vi "Sub Super Duper_7_26_12a_JW.vi"(0 "VISA resource name":refnum<visa-resource-name>="GPIB0::17::INSTR", 1 "Sample Properties:":T6 {"Date Created" format="%<%Y/%m/%d>T"}, 2 "TRF Cluster":T7={"Step 4"=-38.0, "# of Loops"=1.0, "Transfer 2"=FALSE, "Start 4"=-2.0, "Total Points 2"=2, "Start 3"=40.0, "Stop 2"=-40.0, "Step 3"=-1.0, "Loop Step"=0.0, "Integration Time 3"=0, "Loop Wait"=0.0, "First Step"=0.0} {"Loop Wait" format="%<%H:%M:%S>t"; "Integration Time 3" scale=0.0..2.0; "Step 3" format="%.2f"; "Stop 2" format="%.2f"; "Start 3" format="%.2f"; "Start 4" format="%.2f"; "Step 4" format="%.2f"}, 3 "TSP Cluster":T8={"Transport"=FALSE, "Start 2"=0.0, "Stop 3"=-60.0, "Step 2"=-1.0, "Start"=0.0, "Step"=-10.0, "Total Points"=7, "Integration Time"=0} {"Integration Time" scale=0.0..2.0; "Step" format="%.2f"; "Start" format="%.2f"; "Step 2" format="%.2f"; "Stop 3" format="%.2f"; "Start 2" format="%.2f"}, 4 "Compliance Cluster":T3={"Var1 sweep settings"={"sweep spacing (linear: 0)"=0, "sweep mode"=FALSE, "compliance (V)"=100.0, "compliance (A)"=0.001}, "Var1 sweep settings 2"={"sweep spacing (linear: 0)"=0, "sweep mode"=FALSE, "compliance (V)"=100.0, "compliance (A)"=0.001}, "Var2 step settings 2"={"compliance (A)"=0.001, "compliance (V)"=100.0}, "Var2 step settings"={"compliance (A)"=0.001, "compliance (V)"=100.0}} {"Var2 step settings"."compliance (V)" format="%.2f"; "Var2 step settings"."compliance (A)" format="%^.2e"; "Var2 step settings 2"."compliance (V)" format="%.2f"; "Var2 step settings 2"."compliance (A)" format="%^.2e"; "Var1 sweep settings 2"."compliance (A)" format="%^.2e"; "Var1 sweep settings 2"."compliance (V)" format="%.2f"; "Var1 sweep settings 2"."sweep spacing (linear: 0)" items=["linear", "log 10", "log 25", "log 50"]; "Var1 sweep settings"."compliance (A)" format="%^.2e"; "Var1 sweep settings"."compliance (V)" format="%.2f"; "Var1 sweep settings"."sweep spacing (linear: 0)" items=["linear", "log 10", "log 25", "log 50"]}, 5 "error in":errorcluster, 6 "Saved Folder:":path=path "C:/1DATA/2011", 7 "Wait Cluster":T2 {"Wait Time (s)" format="%.1g"; "Wait Countdown" format="%<%H:%M:%S%1u>t"}, 9 "Stop \nCountdown":bool, 11 "Loop Count":dbl) -> (8 "Status Indicator":bool, 10 "Vt Cluster":T1 {"Id Max" format="%.3g"; "Vt Max" format="%.3g"; "Vt Min" format="%.3g"; "Vt Ratio" format="%.3g"}, 13 "Raw Graph":cluster{dbl[], dbl[]}[](graph), 14 "VISA resource name out":refnum<visa-resource-name>, 15 "TRF Path":path, 16 "TSP Path":path, 17 "Graph Cluster":T4, 18 "Char Cluster":T5 {"Mobility-Lin" format="%#_4e"; "On/Off" format="%#_4e"; "Mobility-Sat" format="%#_4e"}, 19 "error out":errorcluster)   [LabVIEW 2011]
uses:
  <vilib>/Platform/TimedLoop/XDataNode/wakeup.ctl
  <vilib>/Platform/TimedLoop/XDataNode/XDNodeRunTimeDep.lvlib
  <vilib>/Platform/TimedLoop/XDataNode/nitl_modes.ctl
  <vilib>/Platform/TimedLoop/XDataNode/timing_clust.ctl
  <vilib>/Platform/TimedLoop/XDataNode/XDataNode.xnode
panel:
  in  "Transport Temp":cluster{"trace":dbl[], "trace":dbl[]}(graph)
  in  "Graph":cluster{dbl[], "trace":dbl[]}[](graph) caption="Transfer"
  # "Vg Sweep"
  # "Vd Step"
  # "Loops and Integration Time"
  # "Device Characteristics"
  # "Sample Properties:"
  # "%"
  # "nm"
  # "Device Properties:"
  # "um"
  # "um"
  # "Vg Step"
  # "Vd Step"
  # "Integration Time"
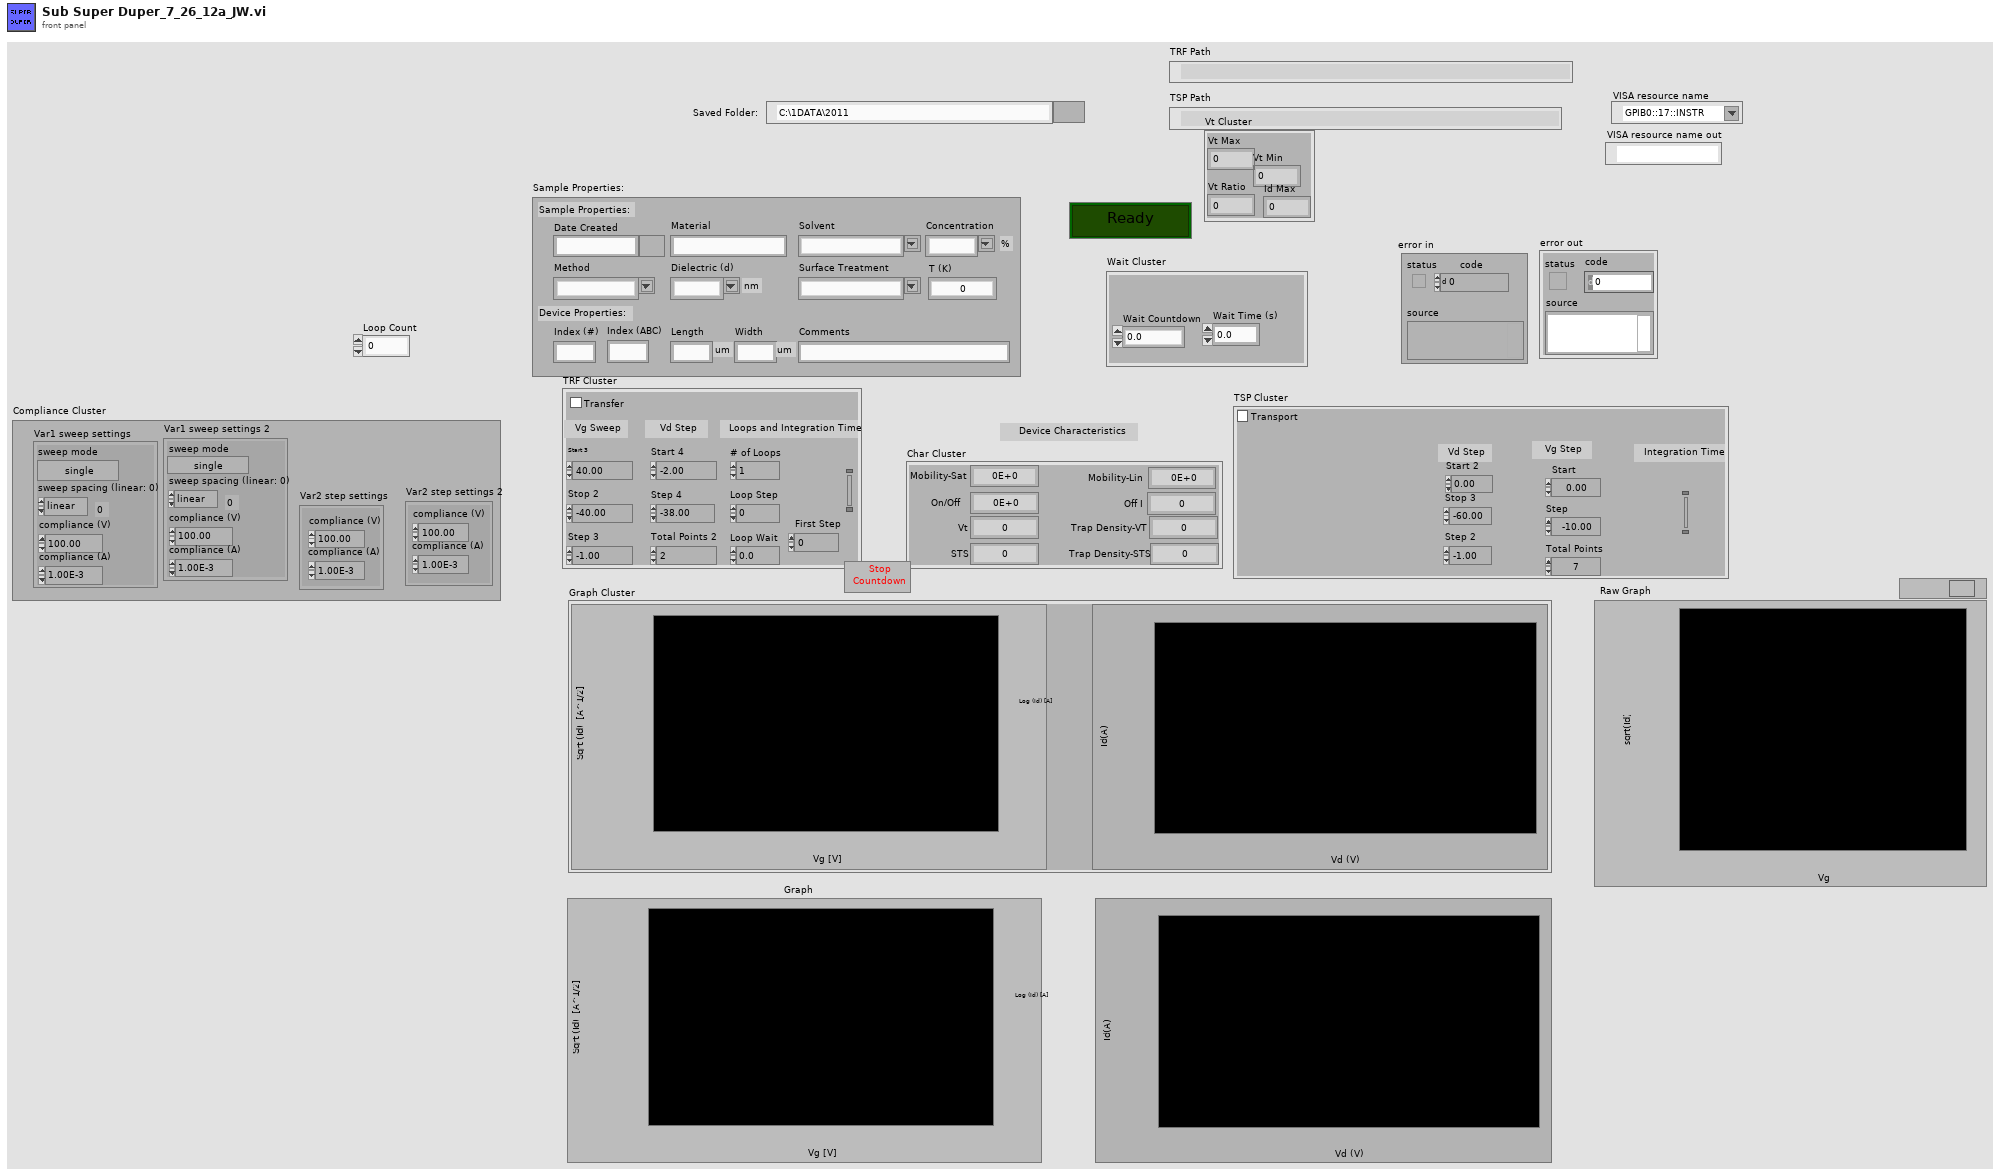
[diagram p1: front panel]
types:
  T1 = cluster{"Vt Max":i32, "Vt Min":i32, "Vt Ratio":i32, "Id Max":i32}
  T2 = cluster{"Wait Countdown":dbl, "Wait Time (s)":dbl}
  T3 = cluster{"Var1 sweep settings":cluster{"sweep spacing (linear: 0)":u16, "sweep mode":bool, "compliance (V)":dbl, "compliance (A)":dbl}, "Var1 sweep settings 2":cluster{"sweep spacing (linear: 0)":u16, "sweep mode":bool, "compliance (V)":dbl, "compliance (A)":dbl}, "Var2 step settings 2":cluster{"compliance (A)":dbl, "compliance (V)":dbl}, "Var2 step settings":cluster{"compliance (A)":dbl, "compliance (V)":dbl}}
  T4 = cluster{"Transfer":cluster{dbl[], "trace":dbl[]}[], "Transport":cluster{"trace":dbl[], "trace":dbl[]}}
  T5 = cluster{"Mobility-Sat":dbl, "Mobility-Lin":dbl, "On/Off ":dbl, "Off I":dbl, "Vt":dbl, "STS":dbl, "Trap Density-VT":dbl, "Trap Density-STS":dbl}
  T6 = cluster{"Date Created":timestamp, "Material":string, "Solvent":string, "Concentration":string, "Method":string, "Dielectric (d)":string, "Index (#)":string, "Index (ABC)":string, "Length":string, "Width":string, "Surface Treatment":string, "Comments":string, "T (K)":dbl}
  T7 = cluster{"Step 4":dbl, "# of Loops":dbl, "Transfer 2":bool, "Start 4":dbl, "Total Points 2":u16, "Start 3":dbl, "Stop 2":dbl, "Step 3":dbl, "Loop Step":dbl, "Integration Time 3":u32, "Loop Wait":dbl, "First Step":dbl}
  T8 = cluster{"Transport":bool, "Start 2":dbl, "Stop 3":dbl, "Step 2":dbl, "Start":dbl, "Step":dbl, "Total Points":u16, "Integration Time":u32}
  T9 = typedef "XDNodeRunTimeDep.lvlib/timing_clust.ctl" = cluster{"Expected End [f-1]":u64, "Actual End [f-1]":u64, "Finished Late? [f-1]":bool, "Expected End [i-1]":u64, "Actual End [i-1]":u64, "Finished Late? [i-1]":bool, "Expected Start [i]":u64, "Actual Start [i]":u64, "Expected Start [f]":u64, "Actual Start [f]":u64, "Source Name":string, "Structure Name":string, "Period":i64, "Deadline":i64, "Offset":i64, "Start":i64, "Priority":i32, "Timeout":i32, "Mode":T10, "Wakeup Reason":T11, "Error":errorcluster, "Source Type":string, "Secondary Source Type":string, "Global End Time":u64, "Global Start Time":u64, "Frame Duration":u64, "Iteration Duration":u64, "Assigned CPU":i32, "I/O Scan Engine Mode":u32}
  T10 = typedef "XDNodeRunTimeDep.lvlib/nitl_modes.ctl" = enum32{"No Change", "Process missed periods, maintain original phase", "Discard missed periods, maintain original phase", "Process missed periods, ignore original phase", "Discard missed periods, ignore original phase"}
  T11 = typedef "XDNodeRunTimeDep.lvlib/wakeup.ctl" = enum32{"Normal", "Aborted", "Asynchronous wakeup", "Timing source error", "Timed loop error", "Timeout"}
  T12 = cluster{"sweep spacing (linear: 0)":u16, "sweep mode":bool, "compliance (V)":dbl, "compliance (A)":dbl}
  T13 = cluster{"compliance (A)":dbl, "compliance (V)":dbl}
  T14 = cluster{"Start 3":dbl, "Stop 2":dbl, "Step 3":dbl, "sweep spacing (linear: 0)":u16, "sweep mode":bool, "compliance (V)":dbl, "compliance (A)":dbl}
  T15 = cluster{"compliance (A)":dbl, "compliance (V)":dbl, "Start 4":dbl, "Total Points 2":u16, dbl}
  T16 = cluster{"Vt Max":i32, "Vt Min":i32, "Vt Ratio":i32, "Id Max":dbl}
  T17 = cluster{"Mobility-Sat":dbl, "Mobility-Lin":dbl, "On/Off Current":dbl, "Off I":dbl, "Vt":dbl, "STS":dbl, "Trap Density-VT":dbl, "Trap Density-STS":dbl}
  T18 = cluster{"Start 2":dbl, "Stop 3":dbl, "Step 2":dbl, "sweep spacing (linear: 0)":u16, "sweep mode":bool, "compliance (V)":dbl, "compliance (A)":dbl}
  T19 = cluster{"compliance (A)":dbl, "compliance (V)":dbl, "Start":dbl, "Total Points":u16, "Step":dbl}
  T20 = cluster{"Graph":cluster{dbl[], "trace":dbl[]}[], "Transport Temp":cluster{"trace":dbl[], "trace":dbl[]}}
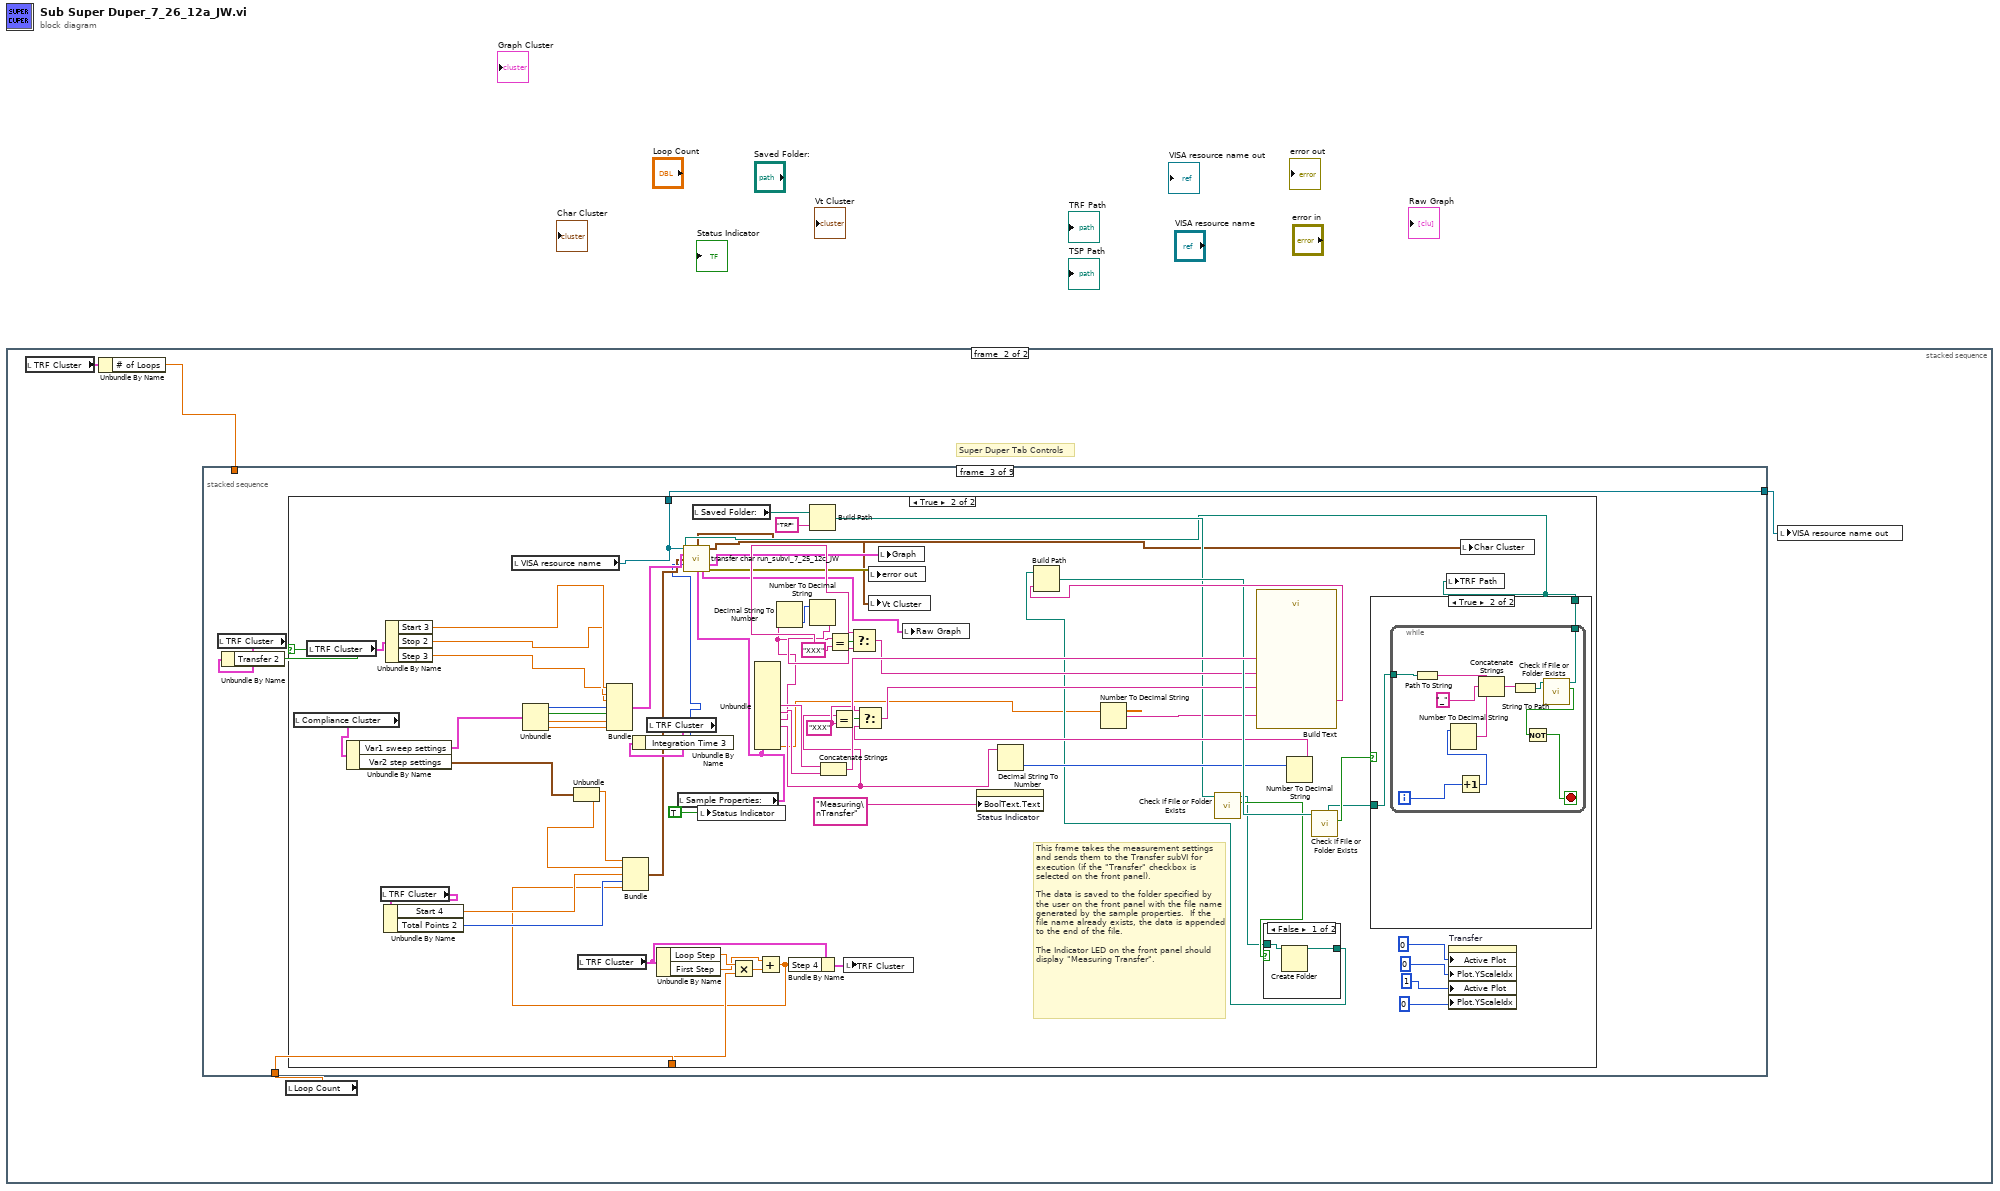
[diagram p0: block diagram]
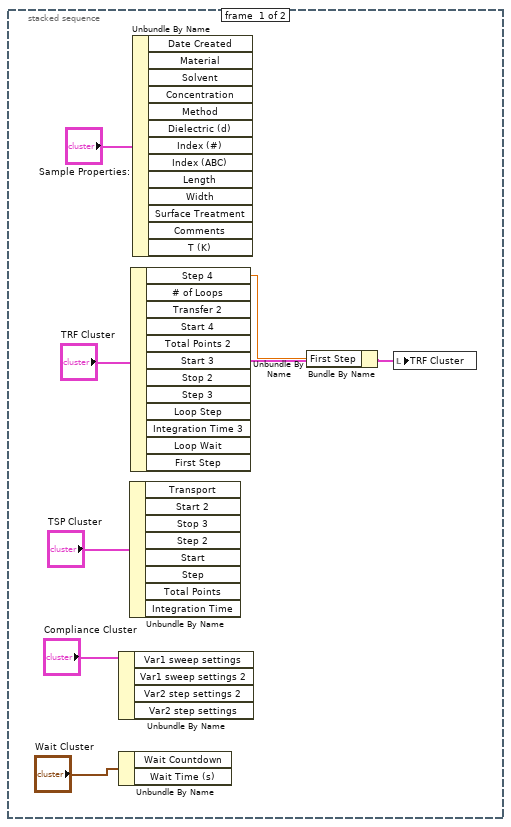
[diagram p2: hidden frame]
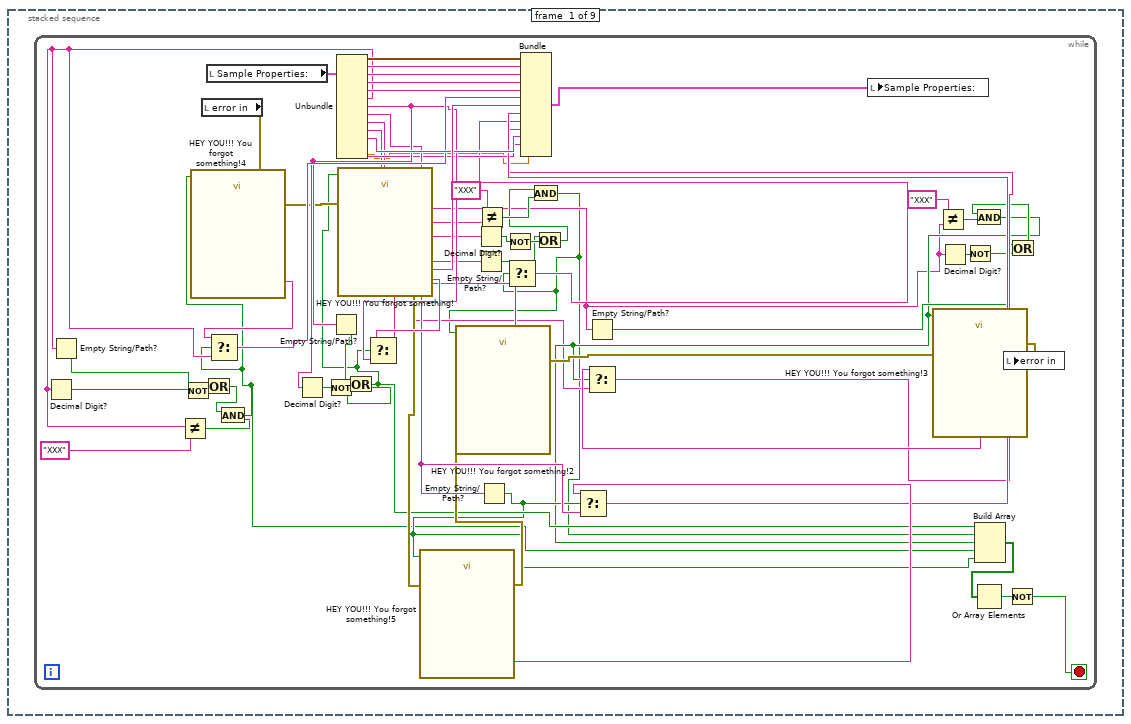
[diagram p3: hidden frame]
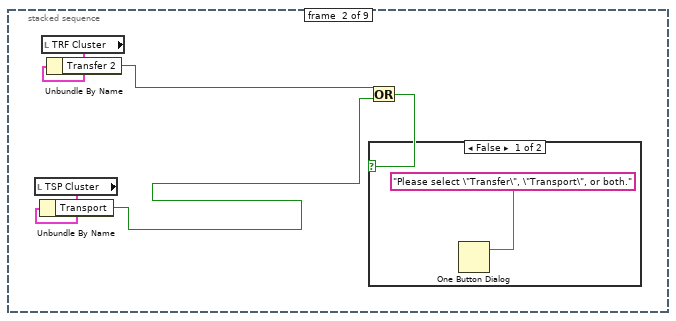
[diagram p4: hidden frame]
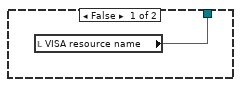
[diagram p6: hidden frame]
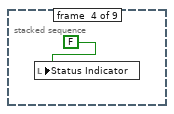
[diagram p9: hidden frame]
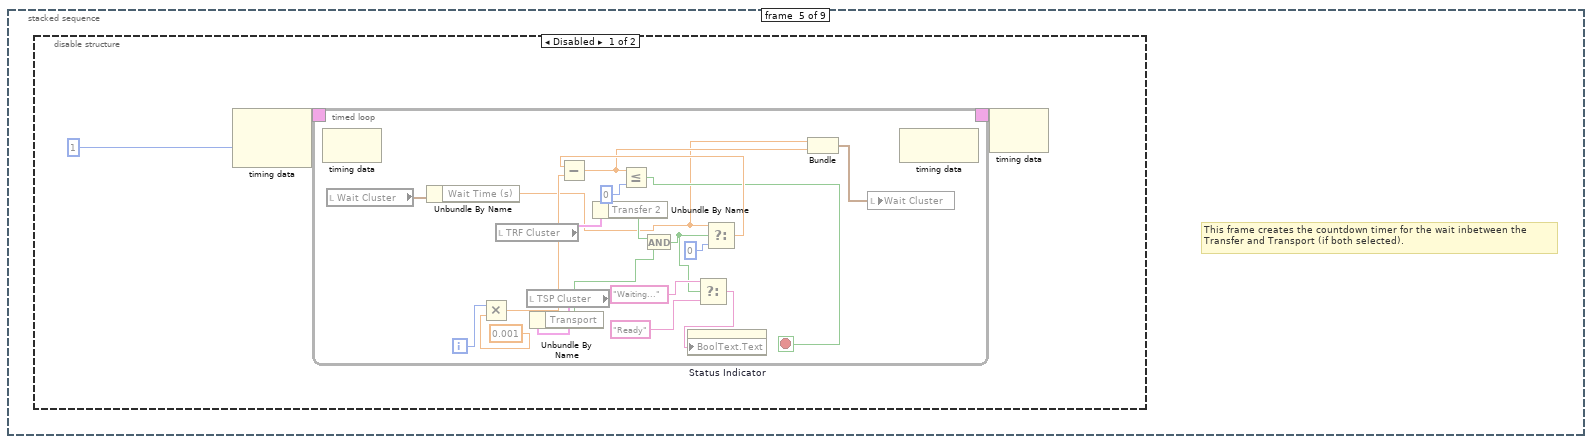
[diagram p10: hidden frame]
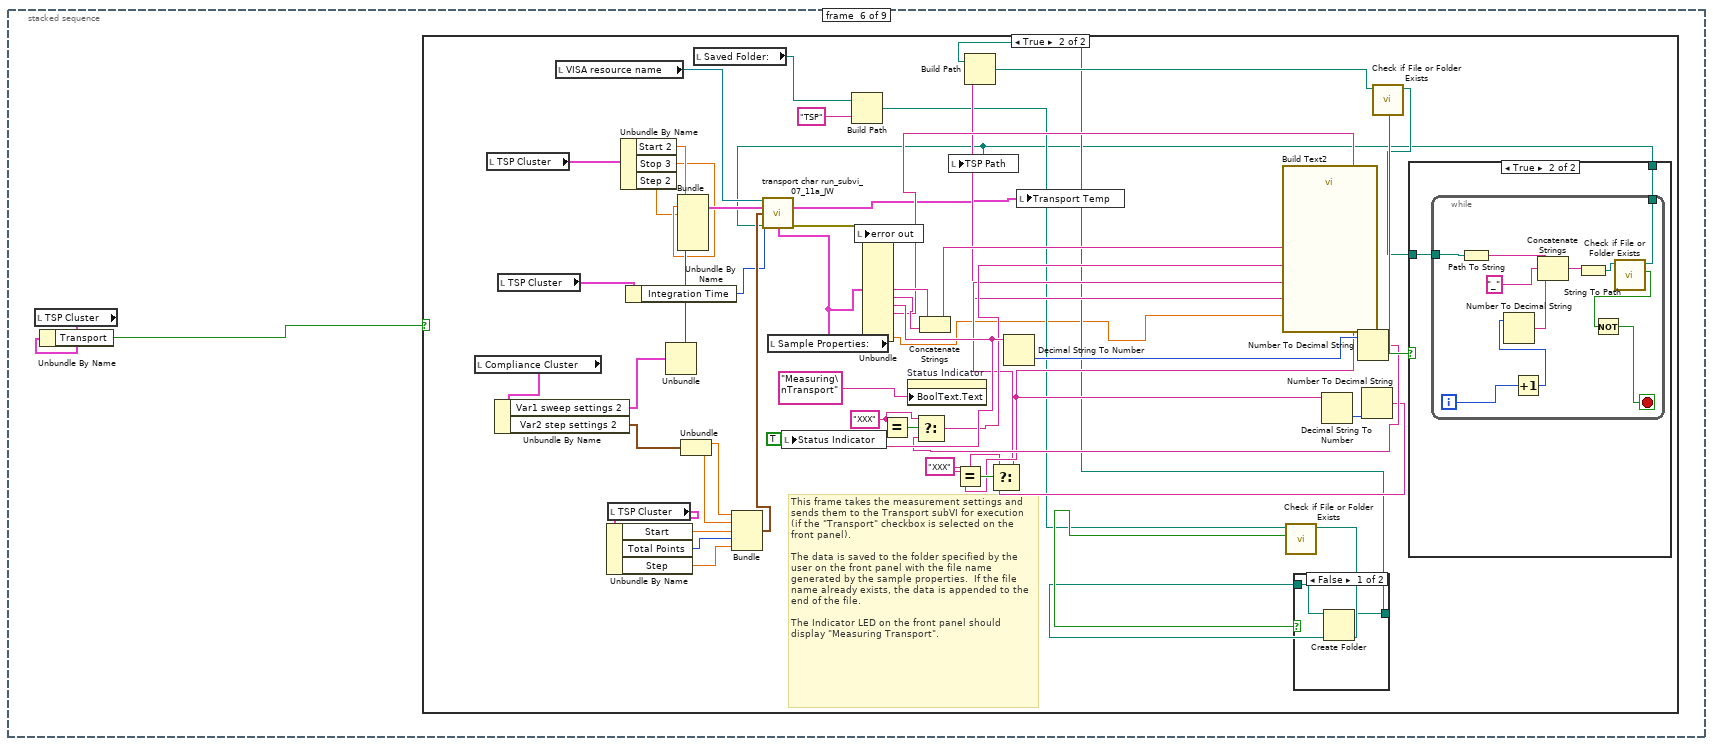
[diagram p12: hidden frame]
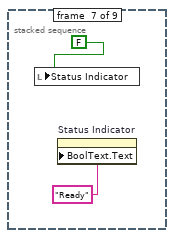
[diagram p16: hidden frame]
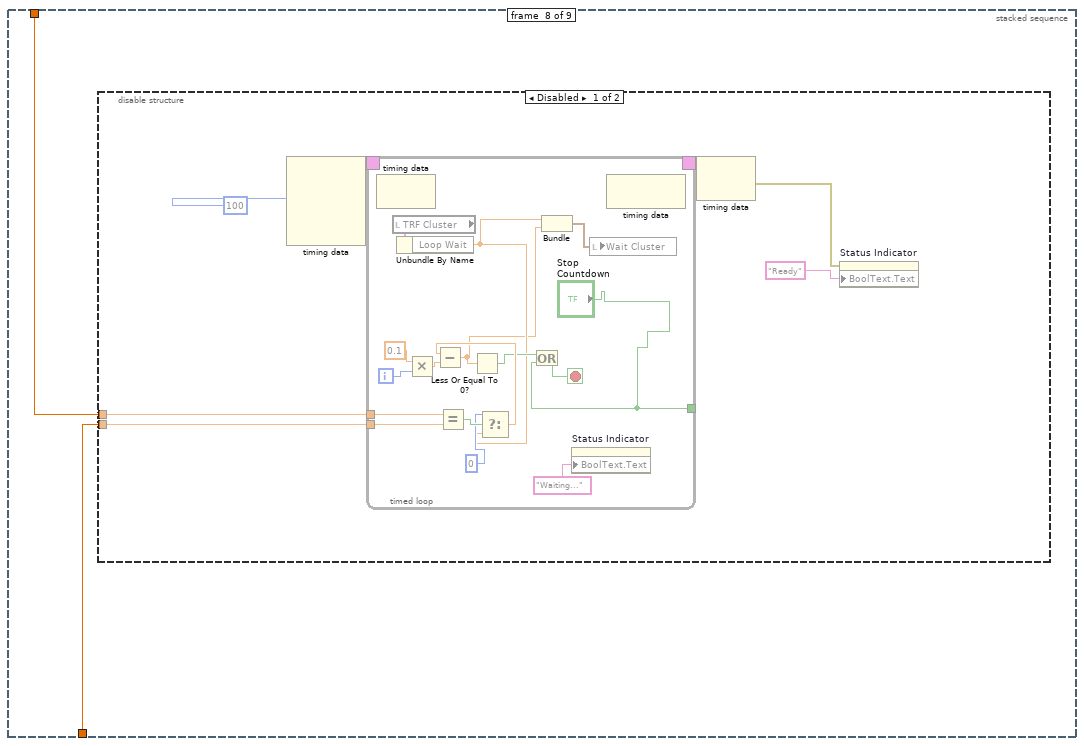
[diagram p17: hidden frame]
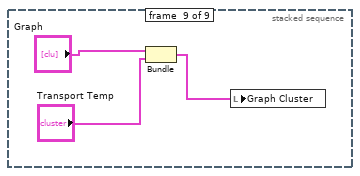
[diagram p19: hidden frame]
diagram:
  n1 = stacked-sequence {
    frame #0 {
      n2 = Unbundle By Name("Compliance Cluster") -> ()  [unwired: 4 out]
      n3 = Unbundle By Name("Wait Cluster") -> ()  [unwired: 2 out]
      n4 = Unbundle By Name("TSP Cluster") -> ()  [unwired: 8 out]
      n5 = Unbundle By Name("TRF Cluster") -> ("Step 4"=w7:dbl)  [unwired: 11 out]
      n6 = Unbundle By Name("Sample Properties:") -> ()  [unwired: 13 out]
      n7 = Bundle By Name(cluster="TRF Cluster", "First Step"=w7) -> (w5:T7)
      n8 = local write "TRF Cluster"(w5) -> ()
    }
    frame #1 {
      # "Super Duper Tab Controls"
      n9 = local read "TRF Cluster"() -> (w11:T7)
      n10 = Unbundle By Name(w11) -> ("# of Loops"=w10:dbl)
      n11 = local read "Loop Count"() -> (w8:dbl)
      n12 = stacked-sequence {
        tunnel: w8 -> [_ _ w81 _ _ _ _ w273 _]
        tunnel: w10 -> [_ _ _ _ _ _ _ w272 _]
        tunnel: [_ _ w78 _ _ _ _ _ _] -> w9
        frame #0 {
          n13 = while {
            stop <- w37 stop-if-true
            n14 = local read "error in"() -> (w43:errorcluster)
            n15 = local read "Sample Properties:"() -> (w66:T6)
            n16 = Unbundle(w66) -> ("Date Created"=w67:timestamp, "Material"=w68:string, "Solvent"=w69:string, "Concentration"=w70:string, "Method"=w71:string, "Dielectric (d)"=w26:string, "Index (#)"=w56:string, "Index (ABC)"=w53:string, "Length"=w21:string, "Width"=w14:string, "Surface Treatment"=w59:string, "Comments"=w51:string, "T (K)"=w12:dbl)
            n17 = Decimal Digit?(1:w26) -> (0:w34:bool)
            n18 = Empty String/Path?(string/path=w26) -> (empty?=w28:bool)
            n19 = Not Equal?(x=w26, y="XXX") -> (x != y?=w25:bool)
            n20 = Not(x=w34) -> (.not. x?=w31:bool)
            n21 = Or(x=w28, y=w31) -> (x .or. y?=w24:bool)
            n22 = And(x=w24, y=w25) -> (x .and. y?=w23:bool)
            n23 = call "HEY YOU!!! You forgot something!4"("Enable"=w23, "error in (no error)"=w43) -> ("Dielectric (d)"=w58:string, "error out"=w42:errorcluster)  [unwired: 15 in, 1 out]
            n24 = Select(t=w58, s=w23, f=w26) -> (s? t:f=w57:string)
            n25 = Decimal Digit?(1:w56) -> (0:w47:bool)
            n26 = Not(x=w47) -> (.not. x?=w46:bool)
            n27 = Empty String/Path?(string/path=w56) -> (empty?=w55:bool)
            n28 = Or(x=w55, y=w46) -> (x .or. y?=w41:bool)
            n29 = call "HEY YOU!!! You forgot something!"("Enable"=w41, "error in (no error)"=w42) -> ("Index (#)"=w65:string, "error out"=w45:errorcluster)  [unwired: 15 in, 1 out]
            n30 = Select(t=w65, s=w41, f=w56) -> (s? t:f=w62:string)
            n31 = Decimal Digit?(1:w21) -> (0:w36:bool)
            n32 = Empty String/Path?(string/path=w21) -> (empty?=w30:bool)
            n33 = Not Equal?(x="XXX", y=w21) -> (x != y?=w20:bool)
            n34 = Empty String/Path?(string/path=w53) -> (empty?=w40:bool)
            n35 = call "HEY YOU!!! You forgot something!5"("Enable"=w40, "error in (no error)"=w45) -> ("Index (ABC)"=w54:string, "error out"=w44:errorcluster)  [unwired: 15 in, 1 out]
            n36 = Not(x=w36) -> (.not. x?=w33:bool)
            n37 = Or(x=w30, y=w33) -> (x .or. y?=w19:bool)
            n38 = And(x=w19, y=w20) -> (x .and. y?=w13:bool)
            n39 = call "HEY YOU!!! You forgot something!2"("Enable"=w13, "error in (no error)"=w44) -> ("Length"=w64:string, "error out"=w61:errorcluster)  [unwired: 15 in, 1 out]
            n40 = Select(t=w64, s=w13, f=w21) -> (s? t:f=w50:string)
            n41 = Select(t=w54, s=w40, f=w53) -> (s? t:f=w52:string)
            n42 = Empty String/Path?(string/path=w14) -> (empty?=w29:bool)
            n43 = Not Equal?(x="XXX", y=w14) -> (x != y?=w18:bool)
            n44 = Decimal Digit?(1:w14) -> (0:w35:bool)
            n45 = Not(x=w35) -> (.not. x?=w32:bool)
            n46 = Or(x=w29, y=w32) -> (x .or. y?=w17:bool)
            n47 = And(x=w17, y=w18) -> (x .and. y?=w16:bool)
            n48 = call "HEY YOU!!! You forgot something!3"("Enable"=w16, "error in (no error)"=w61) -> ("Width"=w63:string, "error out"=w60:errorcluster)  [unwired: 15 in, 1 out]
            n49 = Select(t=w63, s=w16, f=w14) -> (s? t:f=w49:string)
            n50 = Bundle("Date Created"=w67, "Material"=w68, "Solvent"=w69, "Concentration"=w70, "Method"=w71, "Dielectric (d)"=w57, "Index (#)"=w62, "Index (ABC)"=w52, "Length"=w50, "Width"=w49, "Surface Treatment"=w59, "Comments"=w51, "T (K)"=w12) -> (w48:T6)  [unwired: 1 in]
            n51 = local write "Sample Properties:"(w48) -> ()
            n52 = Build Array(w41, w13, w16, w23, w40) -> (w39:bool[])
            n53 = Or Array Elements(Boolean array=w39) -> (logical OR=w38:bool)
            n54 = local write "error in"(w60) -> ()
            n55 = Not(x=w38) -> (.not. x?=w37:bool)
          }
        }
        frame #1 {
          n56 = local read "TSP Cluster"() -> (w73:T8)
          n57 = Unbundle By Name(w73) -> ("Transport"=w72:bool)
          n58 = local read "TRF Cluster"() -> (w75:T7)
          n59 = Unbundle By Name(w75) -> ("Transfer 2"=w74:bool)
          n60 = Or(x=w74, y=w72) -> (x .or. y?=w76:bool)
          n61 = case shown="False" w76 {
            frame False {
              n62 = One Button Dialog(message="Please select \"Transfer\", \"Transport\", or both.") -> ()  [unwired: 1 in, 1 out]
            }
            frame True {
            }
          }
        }
        frame #2 {
          n63 = local read "TRF Cluster"() -> (w79:T7)
          n64 = Unbundle By Name(w79) -> ("Transfer 2"=w80:bool)
          n65 = case shown="True" w80 {
            tunnel: w81 -> [_ w99]
            tunnel: [w82 w93] -> w78
            frame False {
              n66 = local read "VISA resource name"() -> (w82:refnum<visa-resource-name>)
            }
            frame True {
              w128 = "XXX"
              w132 = "XXX"
              # "This frame takes the measurement settings and sends them to the Transfer subVI for execution (if the \"Transfer\" checkbox is selected on the front panel).\n\nThe data is saved to the folder specified by the user on the front panel with the file name generated by the sample properties.  If the file name already exists, the data is appended to the end of the file.\n\nThe Indicator LED on the front panel should display \"Measuring Transfer\"."
              n67 = local read "Compliance Cluster"() -> (w105:T3)
              n68 = local read "TRF Cluster"() -> (w111:T7)
              n69 = Unbundle By Name(w105) -> ("Var1 sweep settings"=w103:T12, "Var2 step settings"=w104:T13)
              n70 = local read "TRF Cluster"() -> (w114:T7)
              n71 = Unbundle By Name(w114) -> ("Start 4"=w113:dbl, "Total Points 2"=w112:u16)
              n72 = Unbundle By Name(w111) -> ("Start 3"=w110:dbl, "Stop 2"=w109:dbl, "Step 3"=w108:dbl)
              n73 = local read "VISA resource name"() -> (w93:refnum<visa-resource-name>)
              n74 = Unbundle(w103) -> ("sweep spacing (linear: 0)"=w150:u16, "sweep mode"=w149:bool, "compliance (V)"=w148:dbl, "compliance (A)"=w147:dbl)
              n75 = Unbundle(w104) -> ("compliance (A)"=w146:dbl, "compliance (V)"=w145:dbl)
              n76 = local read "TRF Cluster"() -> (w94:T7)
              n77 = Bundle("Start 3"=w110, "Stop 2"=w109, "Step 3"=w108, "sweep spacing (linear: 0)"=w150, "sweep mode"=w149, "compliance (V)"=w148, "compliance (A)"=w147) -> (w92:T14)  [unwired: 1 in]
              n78 = local read "TRF Cluster"() -> (w107:T7)
              n79 = Unbundle By Name(w107) -> ("Integration Time 3"=w90:u32)
              n80 = Unbundle By Name(w94) -> ("Loop Step"=w97:dbl, "First Step"=w96:dbl)
              n81 = local read "Sample Properties:"() -> (w88:T6)
              n82 = local read "Saved Folder:"() -> (w106:path)
              n83 = local write "Status Indicator"(TRUE) -> ()
              n84 = Multiply(x=w97, y=w99) -> (x*y=w100:dbl)
              n85 = Unbundle(w88) -> ("Index (#)"=w141:string, "Index (ABC)"=w140:string, "Length"=w124:string, "Width"=w127:string, "T (K)"=w102:dbl)  [unwired: 8 out]
              n86 = Add(x=w96, y=w100) -> (x+y=w95:dbl)
              n87 = Bundle("compliance (A)"=w146, "compliance (V)"=w145, "Start 4"=w113, "Total Points 2"=w112, w95) -> (w91:T15)  [unwired: 1 in]
              n88 = Decimal String To Number(string=w124) -> (number=w135:i32)  [unwired: 2 in, 1 out]
              n89 = Bundle By Name(cluster=w94, "Step 4"=w95) -> (w98:T7)
              n90 = Build Path(base path=w106, name or relative path="TRF") -> (appended path=w120:path)
              n91 = Number To Decimal String(number=w135) -> (decimal integer string=w131:string)  [unwired: 1 in]
              n92 = Concatenate Strings(w141, w140) -> (w139:string)
              n93 = Equal?(x=w124, y=w132) -> (x = y?=w133:bool)
              n94 = Equal?(x=w127, y=w128) -> (x = y?=w129:bool)
              n95 = local write "TRF Cluster"(w98) -> ()
              n96 = Select(t=w132, s=w133, f=w131) -> (s? t:f=w130:string)
              n97 = property on="Status Indicator" class="Bool (strict)"("BoolText.Text"="Measuring\nTransfer") -> ()  [unwired: 2 in, 2 out]
              n98 = Decimal String To Number(string=w127) -> (number=w134:i32)  [unwired: 2 in, 1 out]
              n99 = Number To Decimal String(number=w102) -> (decimal integer string=w101:string)  [unwired: 1 in]
              n100 = call <vilib>:"Check if File or Folder Exists.vi"("path"=w120) -> ("file or folder exists?"=w122:bool, "dup path"=w121:path)  [unwired: 8 in, 1 out]
              n101 = case shown="False" w122 {
                tunnel: w121 -> [w152 w153]
                tunnel: [w151 w153] -> w119
                frame False {
                  n102 = Create Folder(path (use dialog)=w152) -> (created path=w151:path)  [unwired: 2 in, 2 out]
                }
                frame True {
                }
              }
              n103 = Number To Decimal String(number=w134) -> (decimal integer string=w126:string)  [unwired: 1 in]
              n104 = Select(t=w128, s=w129, f=w126) -> (s? t:f=w125:string)
              n105 = call "Build Text"("T"=w101, "Index"=w139, "Length"=w130, "Width"=w125) -> ("Result"=w144:string)  [unwired: 10 in, 1 out]
              n106 = Build Path(base path=w119, name or relative path=w144) -> (appended path=w137:path)
              n107 = call <vilib>:"Check if File or Folder Exists.vi"("path"=w137) -> ("file or folder exists?"=w138:bool, "dup path"=w136:path)  [unwired: 8 in, 1 out]
              n108 = case shown="True" w138 {
                tunnel: w136 -> [w154 w156]
                tunnel: [w154 w155] -> w89
                frame False {
                }
                frame True {
                  n109 = while {
                    tunnel: w156 -> [w158]
                    tunnel: [w157] -> w155
                    i -> [w160]
                    stop <- w161 stop-if-true
                    n110 = Path To String(path=w158) -> (string=w167:string)
                    n111 = Increment(x=w160) -> (x+1=w159:i32)
                    n112 = Number To Decimal String(number=w159) -> (decimal integer string=w165:string)  [unwired: 1 in]
                    n113 = Concatenate Strings(w167, "_", w165) -> (w164:string)
                    n114 = String To Path(string=w164) -> (path=w163:path)
                    n115 = call <vilib>:"Check if File or Folder Exists.vi"("path"=w163) -> ("file or folder exists?"=w162:bool, "dup path"=w157:path)  [unwired: 8 in, 1 out]
                    n116 = Not(x=w162) -> (.not. x?=w161:bool)
                  }
                }
              }
              n117 = call "transfer char run_subvi_7_25_12c_JW.vi"("VISA session"=w93, "Var1 sweep settings"=w92, "Var2 step settings"=w91, "integration time"=w90, "Input Path"=w89, "Sample Properties:"=w88) -> ("Check Cluster"=w84:T16, "Output"=w85:T17, "XY Graph"=w86:cluster{dbl[], "trace":dbl[]}[], "Raw Graph"=w83:cluster{dbl[], dbl[]}[], "error?"=w87:errorcluster)  [unwired: 3 in, 2 out]
              n118 = local write "error out"(w87) -> ()
              n119 = local write "Vt Cluster"(w84) -> ()
              n120 = local write "Graph"(w86) -> ()
              n121 = local write "Raw Graph"(w83) -> ()
              n122 = local write "TRF Path"(w89) -> ()
              n123 = property on="Transfer" class="XYGraph (strict)"("Active Plot"=0, "Plot.YScaleIdx"=0, "Active Plot"=1, "Plot.YScaleIdx"=0) -> ()  [unwired: 2 in, 2 out]
              n124 = local write "Char Cluster"(w85) -> ()
            }
          }
        }
        frame #3 {
          n125 = local write "Status Indicator"(FALSE) -> ()
        }
        frame #4 {
          # "This frame creates the countdown timer for the wait inbetween the\nTransfer and Transport (if both selected)."
          n126 = disable-structure shown="Disabled" {
            frame Disabled {
              n127 = node-c288(1) -> (w171:T9)  [unwired: 1 in]
              n128 = timed-loop {
                timing: w171 -> [_]
                timing-out: [_] -> w170
                i -> [w182]
                stop <- w183 stop-if-true
                n129 = node-c288() -> ()  [unwired: 1 in, 1 out]
                n130 = local read "Wait Cluster"() -> (w175:T2)
                n131 = Unbundle By Name(w175) -> ("Wait Time (s)"=w173:dbl)
                n132 = Multiply(x=w182, y=0.001) -> (x*y=w180:dbl)
                n133 = local read "TRF Cluster"() -> (w176:T7)
                n134 = local read "TSP Cluster"() -> (w177:T8)
                n135 = Unbundle By Name(w177) -> ("Transport"=w178:bool)
                n136 = Unbundle By Name(w176) -> ("Transfer 2"=w179:bool)
                n137 = And(x=w179, y=w178) -> (x .and. y?=w187:bool)
                n138 = Select(t="Waiting...", s=w187, f="Ready") -> (s? t:f=w189:string)
                n139 = property on="Status Indicator" class="Bool (strict)"("BoolText.Text"=w189) -> ()  [unwired: 2 in, 2 out]
                n140 = Select(t=w173, s=w187, f=0) -> (s? t:f=w185:dbl)
                n141 = Subtract(x=w185, y=w180) -> (x-y=w174:dbl)
                n142 = Less Or Equal?(x=w174, y=0) -> (x <= y?=w183:bool)
                n143 = Bundle("Wait Time (s)"=w173, w174) -> (w172:cluster{"Wait Time (s)":dbl, dbl})  [unwired: 1 in]
                n144 = local write "Wait Cluster"(w172) -> ()
                n145 = node-c288() -> ()  [unwired: 1 in, 1 out]
              }
              n146 = node-c288(w170) -> ()  [unwired: 1 out]
            }
            frame Enabled {
            }
          }
        }
        frame #5 {
          n147 = local read "TSP Cluster"() -> (w198:T8)
          n148 = Unbundle By Name(w198) -> ("Transport"=w197:bool)
          n149 = case shown="True" w197 {
            frame False {
            }
            frame True {
              w225 = "XXX"
              w229 = "XXX"
              # "This frame takes the measurement settings and sends them to the Transport subVI for execution (if the \"Transport\" checkbox is selected on the front panel).\n\nThe data is saved to the folder specified by the user on the front panel with the file name generated by the sample properties.  If the file name already exists, the data is appended to the end of the file.\n\nThe Indicator LED on the front panel should display \"Measuring Transport\"."
              n150 = local read "Compliance Cluster"() -> (w203:T3)
              n151 = local read "TSP Cluster"() -> (w216:T8)
              n152 = Unbundle By Name(w203) -> ("Var1 sweep settings 2"=w202:T12, "Var2 step settings 2"=w201:T13)
              n153 = local read "TSP Cluster"() -> (w209:T8)
              n154 = local read "VISA resource name"() -> (w205:refnum<visa-resource-name>)
              n155 = local read "TSP Cluster"() -> (w207:T8)
              n156 = Unbundle By Name(w207) -> ("Start"=w212:dbl, "Total Points"=w211:u16, "Step"=w210:dbl)
              n157 = Unbundle By Name(w216) -> ("Start 2"=w215:dbl, "Stop 3"=w214:dbl, "Step 2"=w213:dbl)
              n158 = Unbundle By Name(w209) -> ("Integration Time"=w208:u32)
              n159 = Unbundle(w202) -> ("sweep spacing (linear: 0)"=w252:u16, "sweep mode"=w251:bool, "compliance (V)"=w250:dbl, "compliance (A)"=w249:dbl)
              n160 = Bundle("Start 2"=w215, "Stop 3"=w214, "Step 2"=w213, "sweep spacing (linear: 0)"=w252, "sweep mode"=w251, "compliance (V)"=w250, "compliance (A)"=w249) -> (w248:T18)  [unwired: 1 in]
              n161 = Unbundle(w201) -> ("compliance (A)"=w247:dbl, "compliance (V)"=w246:dbl)
              n162 = local read "Saved Folder:"() -> (w204:path)
              n163 = Bundle("compliance (A)"=w247, "compliance (V)"=w246, "Start"=w212, "Total Points"=w211, "Step"=w210) -> (w245:T19)  [unwired: 1 in]
              n164 = local read "Sample Properties:"() -> (w241:T6)
              n165 = local write "Status Indicator"(TRUE) -> ()
              n166 = Build Path(base path=w204, name or relative path="TSP") -> (appended path=w218:path)
              n167 = Unbundle(w241) -> ("Index (#)"=w240:string, "Index (ABC)"=w239:string, "Length"=w230:string, "Width"=w226:string, "T (K)"=w199:dbl)  [unwired: 8 out]
              n168 = Equal?(x=w229, y=w230) -> (x = y?=w231:bool)
              n169 = property on="Status Indicator" class="Bool (strict)"("BoolText.Text"="Measuring\nTransport") -> ()  [unwired: 2 in, 2 out]
              n170 = Concatenate Strings(w240, w239) -> (w238:string)
              n171 = Equal?(x=w225, y=w226) -> (x = y?=w234:bool)
              n172 = Decimal String To Number(string=w230) -> (number=w233:i32)  [unwired: 2 in, 1 out]
              n173 = call <vilib>:"Check if File or Folder Exists.vi"("path"=w218) -> ("file or folder exists?"=w220:bool, "dup path"=w219:path)  [unwired: 8 in, 1 out]
              n174 = case shown="False" w220 {
                tunnel: w219 -> [w254 w255]
                tunnel: [w253 w255] -> w217
                frame False {
                  n175 = Create Folder(path (use dialog)=w254) -> (created path=w253:path)  [unwired: 2 in, 2 out]
                }
                frame True {
                }
              }
              n176 = Decimal String To Number(string=w226) -> (number=w232:i32)  [unwired: 2 in, 1 out]
              n177 = Number To Decimal String(number=w233) -> (decimal integer string=w228:string)  [unwired: 1 in]
              n178 = Select(t=w229, s=w231, f=w228) -> (s? t:f=w227:string)
              n179 = Number To Decimal String(number=w232) -> (decimal integer string=w224:string)  [unwired: 1 in]
              n180 = Select(t=w225, s=w234, f=w224) -> (s? t:f=w223:string)
              n181 = call "Build Text2"("T"=w199, "Index"=w238, "Length"=w227, "Width"=w223) -> ("Result"=w222:string)  [unwired: 10 in, 1 out]
              n182 = Build Path(base path=w217, name or relative path=w222) -> (appended path=w235:path)
              n183 = call <vilib>:"Check if File or Folder Exists.vi"("path"=w235) -> ("file or folder exists?"=w237:bool, "dup path"=w236:path)  [unwired: 8 in, 1 out]
              n184 = case shown="True" w237 {
                tunnel: w236 -> [w256 w258]
                tunnel: [w256 w257] -> w200
                frame False {
                }
                frame True {
                  n185 = while {
                    tunnel: w258 -> [w260]
                    tunnel: [w259] -> w257
                    i -> [w262]
                    stop <- w263 stop-if-true
                    n186 = Path To String(path=w260) -> (string=w269:string)
                    n187 = Increment(x=w262) -> (x+1=w261:i32)
                    n188 = Number To Decimal String(number=w261) -> (decimal integer string=w267:string)  [unwired: 1 in]
                    n189 = Concatenate Strings(w269, "_", w267) -> (w266:string)
                    n190 = String To Path(string=w266) -> (path=w265:path)
                    n191 = call <vilib>:"Check if File or Folder Exists.vi"("path"=w265) -> ("file or folder exists?"=w264:bool, "dup path"=w259:path)  [unwired: 8 in, 1 out]
                    n192 = Not(x=w264) -> (.not. x?=w263:bool)
                  }
                }
              }
              n193 = call "transport char run_subvi_07_11a_JW.vi"("VISA session"=w205, "Var1 sweep settings"=w248, "Var2 step settings"=w245, "integration time"=w208, "Path"=w200, "Sample Properties:"=w241) -> ("graphic display"=w206:cluster{"trace":dbl[], "trace":dbl[]}, "error?"=w244:errorcluster)  [unwired: 8 in]
              n194 = local write "error out"(w244) -> ()
              n195 = local write "TSP Path"(w200) -> ()
              n196 = local write "Transport Temp"(w206) -> ()
            }
          }
        }
        frame #6 {
          n197 = local write "Status Indicator"(FALSE) -> ()
          n198 = property on="Status Indicator" class="Bool (strict)"("BoolText.Text"="Ready") -> ()  [unwired: 2 in, 2 out]
        }
        frame #7 {
          n199 = disable-structure shown="Disabled" {
            disable-tunnel: w273 -> [w275 _]
            disable-tunnel: w272 -> [w274 _]
            frame Disabled {
              n200 = node-c288(100) -> (w280:T9)  [unwired: 3 in]
              n201 = timed-loop {
                timing: w280 -> [_]
                timing-out: [_] -> w279
                tunnel: w275 -> [w291]
                tunnel: w274 -> [w290]
                tunnel: ["Stop \nCountdown"] -> _
                i -> [w296]
                stop <- w286 stop-if-true
                n202 = node-c288() -> ()  [unwired: 1 in, 1 out]
                n203 = local read "TRF Cluster"() -> (w285:T7)
                n204 = Unbundle By Name(w285) -> ("Loop Wait"=w283:dbl)
                n205 = Multiply(x=0.1, y=w296) -> (x*y=w294:dbl)
                n206 = Equal?(x=w290, y=w291) -> (x = y?=w292:bool)
                n207 = Select(t=0, s=w292, f=w283) -> (s? t:f=w288:dbl)
                n208 = Subtract(x=w288, y=w294) -> (x-y=w282:dbl)
                n209 = Less Or Equal To 0?(x=w282) -> (x <= 0?=w287:bool)
                n210 = Or(x=w287, y="Stop \nCountdown") -> (x .or. y?=w286:bool)
                n211 = Bundle("Loop Wait"=w283, w282) -> (w284:cluster{"Loop Wait":dbl, dbl})  [unwired: 1 in]
                n212 = property on="Status Indicator" class="Bool (strict)"("BoolText.Text"="Waiting...") -> ()  [unwired: 2 in, 2 out]
                n213 = local write "Wait Cluster"(w284) -> ()
                n214 = node-c288() -> ()  [unwired: 1 in, 1 out]
              }
              n215 = node-c288(w279) -> (w276:errorcluster)
              n216 = property on="Status Indicator" class="Bool (strict)"(error in=w276, "BoolText.Text"="Ready") -> ()  [unwired: 1 in, 2 out]
            }
            frame Enabled {
            }
          }
        }
        frame #8 {
          n217 = Bundle("Graph"="Graph", "Transport Temp"="Transport Temp") -> (w306:T20)  [unwired: 1 in]
          n218 = local write "Graph Cluster"(w306) -> ()
        }
      }
      n219 = local write "VISA resource name out"(w9) -> ()
    }
  }
